vi "Update Routing Channel Description.vi"(8 "error in (no error)":errorcluster, 10 "New Description":string, 11 "Channel Ref in":T1 format="%.0x") -> (0 "error out":errorcluster, 3 "Channel Ref out":T1 format="%.0x")   [LabVIEW 2017, in "SLSC Switch Scripting.lvlib"]
uses:
  SLSC Switch Scripting.lvlib
  <vilib>/NI Veristand/Custom Device API/Custom Device Item Ref.ctl
  <vilib>/NI VeriStand/Custom Device API/Custom Device API.lvlib
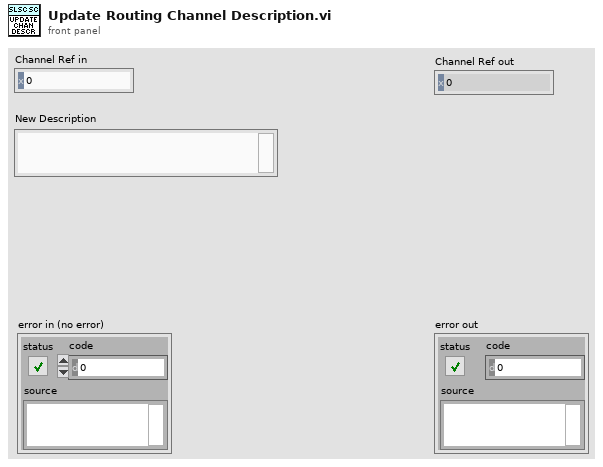
[diagram p1: front panel]
types:
  T1 = typedef "Custom Device API.lvlib/Custom Device Item Ref.ctl" = u64
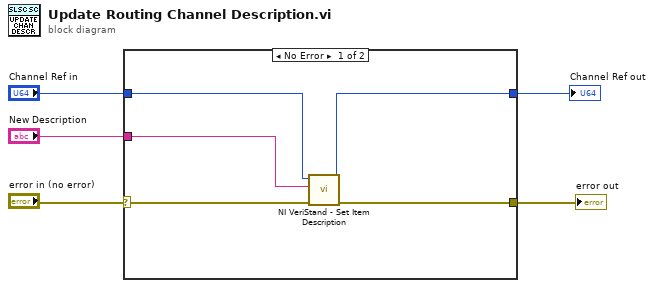
[diagram p0: block diagram]
diagram:
  n1 = case shown="No Error" "error in (no error)" {
    selector: "error in (no error)" -> [w6 w12]
    tunnel: [w8 w12] -> w1
    tunnel: [w9 w11] -> w2
    tunnel: "Channel Ref in" -> [w10 w11]
    tunnel: "New Description" -> [w7 _]
    frame No Error {
      n2 = call <vilib>:"NI VeriStand - Set Item Description.vi"("error in (no error)"=w6, "Description"=w7, "Item Ref in"=w10) -> ("error out"=w8:errorcluster, "Item Ref out"=w9:T1)  [unwired: 6 in, 1 out]
    }
    frame Error {
    }
  }
  "error out" <- w1
  "Channel Ref out" <- w2
